vi "Write Notes.vi"(8 "error in (no error)":errorcluster, 10 "Notes":string, 11 "Data Save":refnum<class "LV-Data.lvclass">) -> (0 "error out":errorcluster, 3 "Data Save out":refnum<class "LV-Data.lvclass">)   [LabVIEW 2019, in "LV-Data.lvclass"]
uses:
  LV-Data.lvclass
  LV-Data.lvclass/LV-Data.ctl
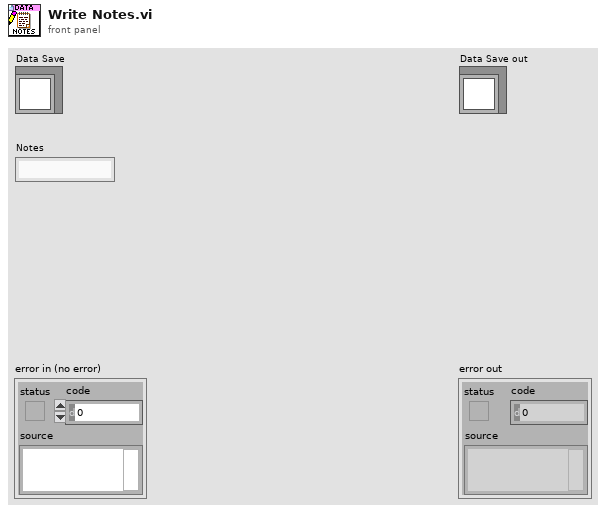
[diagram p1: front panel]
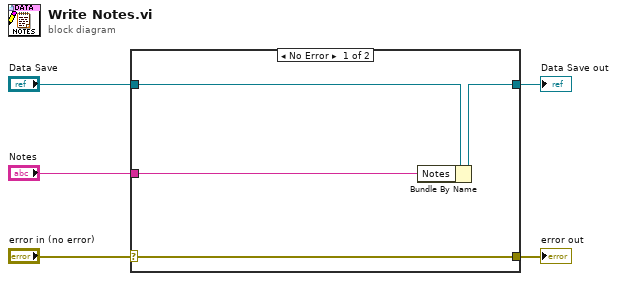
[diagram p0: block diagram]
diagram:
  n1 = case shown="No Error" "error in (no error)" {
    selector: "error in (no error)" -> [w9 w10]
    tunnel: [w9 w10] -> w4
    tunnel: [w6 w11] -> w2
    tunnel: "Data Save" -> [w8 w11]
    tunnel: "Notes" -> [w7 _]
    frame No Error {
      n2 = Bundle By Name(cluster=w8, "Notes"=w7) -> (w6:refnum<class "LV-Data.lvclass">)
    }
    frame Error {
    }
  }
  "error out" <- w4
  "Data Save out" <- w2
